vi "Scan_Format.vi"(1 "字符串格式(%.6f)":string="%.6f", 2 "要转化的数字":dbl, 3 "数字标题":string, 4 "原始字符串":string) -> (0 "输出转换结果":string)   [LabVIEW 2020]
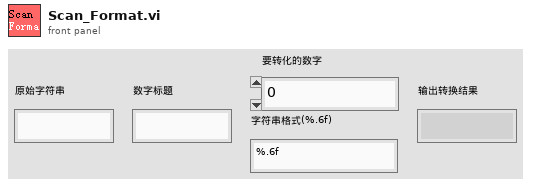
[diagram p1: front panel]
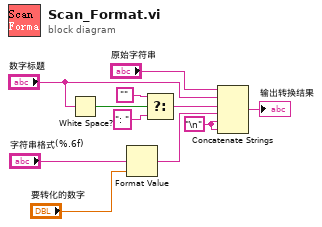
[diagram p0: block diagram]
diagram:
  w1 = "\n"
  n1 = White Space?(1:"数字标题") -> (0:w6:bool)
  n2 = Format Value(format string="字符串格式(%.6f)", value (0)="要转化的数字") -> (output string=w9:string)  [unwired: 1 in]
  n3 = Select(t="", s=w6, f=": ") -> (s? t:f=w3:string)
  n4 = Concatenate Strings("原始字符串", "数字标题", w3, w9, w1, w1) -> (→"输出转换结果":string)
